vi "GetCorePaths.vi"() -> (2 "TemplatesPath":path, 3 "LibPath":path)   [LabVIEW 2017]
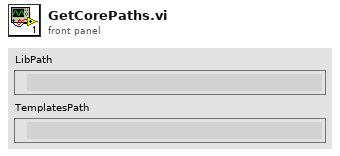
[diagram p1: front panel]
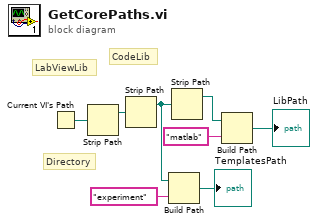
[diagram p0: block diagram]
diagram:
  # "CodeLib"
  # "LabViewLib"
  # "Directory"
  n1 = Current VI's Path() -> (path=w8:path)
  n2 = Strip Path(path=w8) -> (stripped path=w7:path)  [unwired: 1 out]
  n3 = Strip Path(path=w7) -> (stripped path=w6:path)  [unwired: 1 out]
  n4 = Build Path(base path=w6, name or relative path="experiment") -> (appended path=→"TemplatesPath":path)
  n5 = Strip Path(path=w6) -> (stripped path=w2:path)  [unwired: 1 out]
  n6 = Build Path(base path=w2, name or relative path="matlab") -> (appended path=→"LibPath":path)
